vi "PC_main.vi"() -> ()   [LabVIEW 2016]
panel:
  in  "stop":bool
  in  "speed":i32
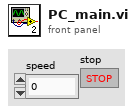
[diagram p1: front panel]
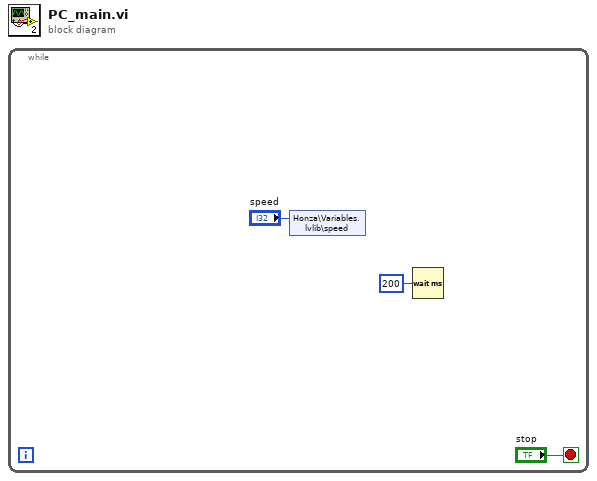
[diagram p0: block diagram]
diagram:
  n1 = while {
    stop <- "stop" stop-if-true
    n2 = shared-variable "Honza\\Variables.lvlib\\speed"("speed") -> ()  [unwired: 1 in, 1 out]
    n3 = Wait (ms)(milliseconds to wait=u32 200) -> ()  [unwired: 1 out]
  }
